vi "poll spawned task.vi"(0 "JSON string in":string, 5 "polling control":T1={"Timeout, ms (-1)"=-1, "polling period (ms)"={"starting"=4, "final"=128}, "interrupt polling notifier"=refnum}, 11 "error in (no error)":errorcluster) -> (3 "timeout?":bool, 4 "JSON received":string, 6 "Notifier out":refnum<notifier>, 8 "done":bool, 10 "Jl Server state out":T2, 12 "detailed error info":T3, 13 "Notification out":bool, 14 "return code":u8, 15 "error out":errorcluster)   [LabVIEW 2018, in "LV2Julia_core.lvlib"]
uses:
  LV2Julia_core.lvlib
  detailed error info.ctl
  StackFrame.ctl
  Server or client state.ctl
  polling control.ctl
  958caf3f-946f-4dc4-9902-e12cbf4cba19.vi
  958caf3f-946f-4dc4-9902-e12cbf4cba19.vi/ee613294-7676-459b-bae0-527ec17cd08f.vi
  958caf3f-946f-4dc4-9902-e12cbf4cba19.vi/ee613294-7676-459b-bae0-527ec17cd08f.vi/324bc100-61cc-4399-8a28-7e417bd8f265.vi
  958caf3f-946f-4dc4-9902-e12cbf4cba19.vi/ee613294-7676-459b-bae0-527ec17cd08f.vi/1a2262df-f044-41fe-b48a-3393a41bf191.vi
  958caf3f-946f-4dc4-9902-e12cbf4cba19.vi/ee613294-7676-459b-bae0-527ec17cd08f.vi/0df26e2a-8cb6-4a42-a810-c7ba34c0704a.vi
  check ID validity.vi
  bindata_descr to JSON.vi
  check cluster field names.vi
  concat JSON.vi
  build request.vi
  REQ full lifecycle.vi
  Parse server response.vi
  log jl exceptions.vi
panel:
  out "parsed response":cluster{"ticket":i32}
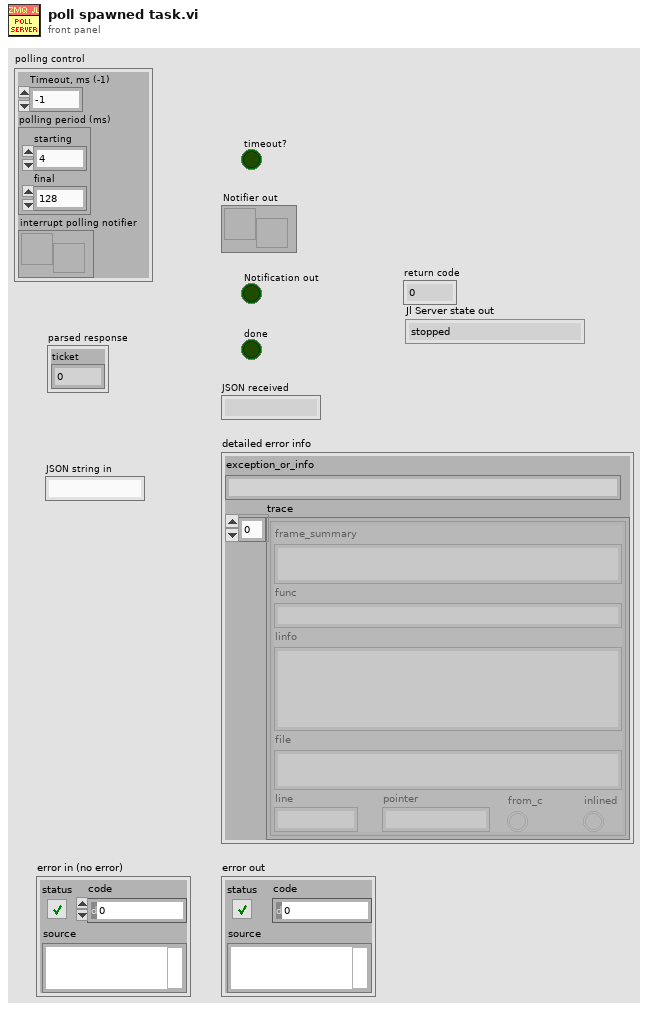
[diagram p1: front panel]
types:
  T1 = typedef "polling control.ctl" = cluster{"Timeout, ms (-1)":i32, "polling period (ms)":cluster{"starting":i32, "final":i32}, "interrupt polling notifier":refnum<notifier>}
  T2 = typedef "LV2Julia_core.lvlib/Server or client state.ctl" = enum16{"stopped", "running", "unknown"}
  T3 = typedef "LV2Julia_core.lvlib/detailed error info.ctl" = cluster{"exception_or_info":string, "trace":T4[]}
  T4 = typedef "LV2Julia_core.lvlib/StackFrame.ctl" = cluster{"frame_summary":string, "func":string, "linfo":string, "file":string, "line":i32, "pointer":u64, "from_c":bool, "inlined":bool}
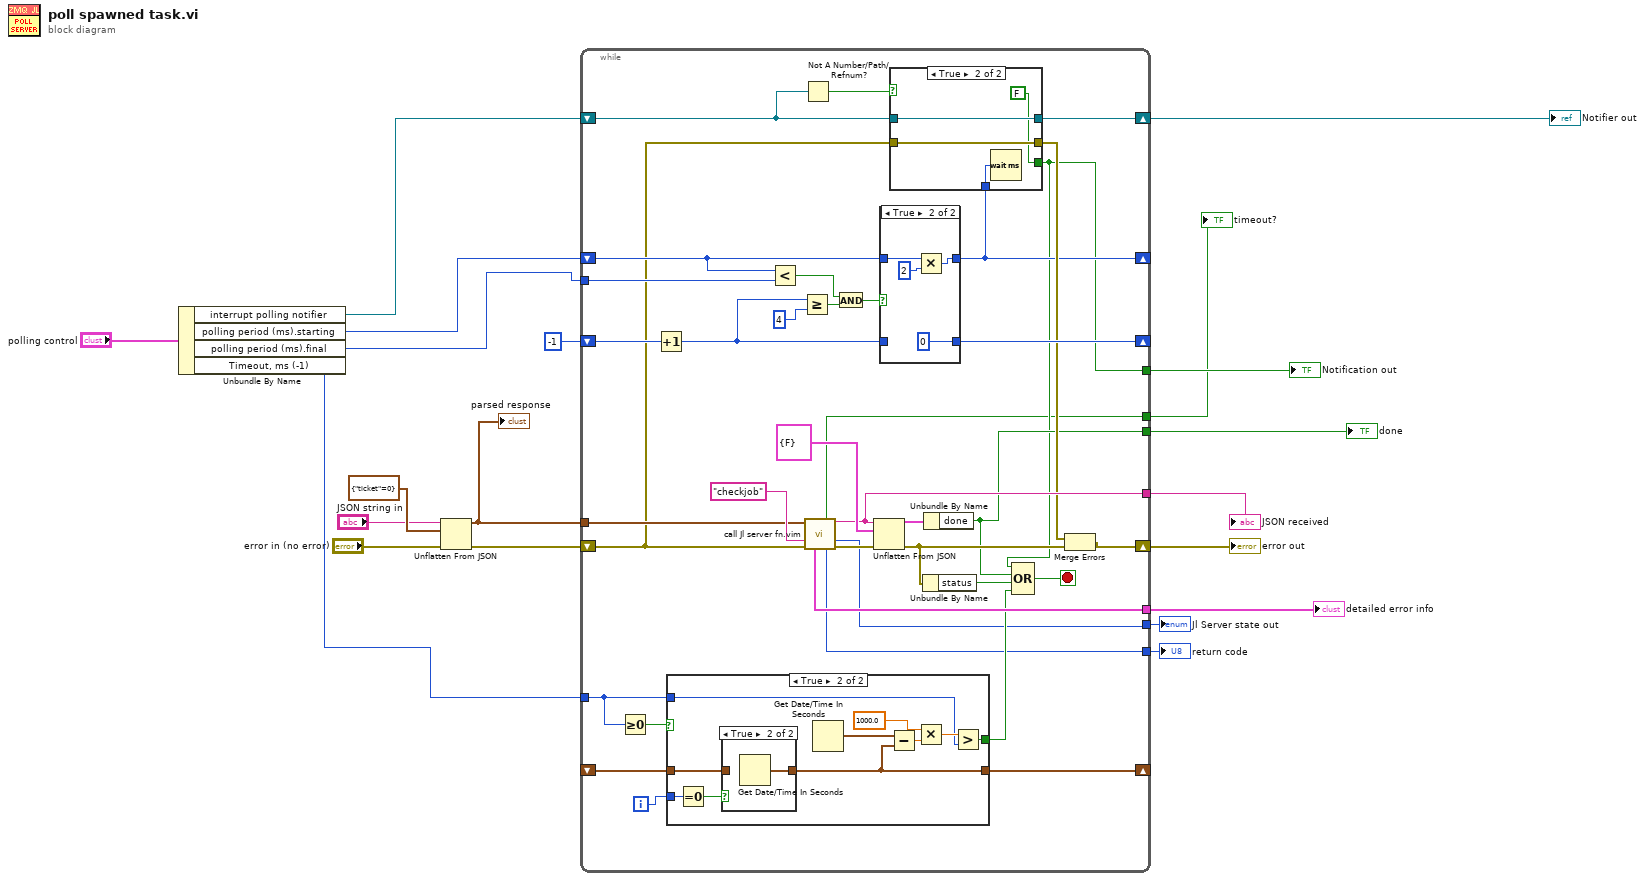
[diagram p0: block diagram]
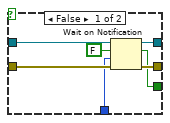
[diagram p2: hidden frame]
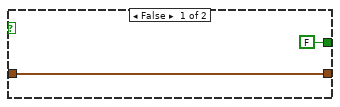
[diagram p3: hidden frame]
diagram:
  n1 = Unbundle By Name("polling control") -> ("interrupt polling notifier"=w1:refnum<notifier>, "polling period (ms).starting"=w3:i32, "polling period (ms).final"=w2:i32, "Timeout, ms (-1)"=w4:i32)
  n2 = Unflatten From JSON(JSON string="JSON string in", type and defaults=cluster{"ticket":i32} {"ticket"=0} ("parsed response"), error in (no error)="error in (no error)") -> (value=w6:cluster{"ticket":i32}, error out=w7:errorcluster)  [unwired: 4 in]
  "parsed response" <- w6
  n3 = while {
    tunnel: w6 -> [w56]
    tunnel: [w52] -> w13
    shift-right: [w38] -> w14
    shift-left: w7 -> [w39]
    shift-right: [w35] -> _
    shift-left: w3 -> [w42]
    shift-right: [w47] -> _
    shift-left: -1 ("counter") -> [w48]
    tunnel: w2 -> [w44]
    shift-right: [w36] -> w16
    shift-left: w1 -> [w21]
    tunnel: [w28] -> w20
    tunnel: w4 -> [w25]
    shift-right: [w30] -> _
    shift-left: _ -> [w33]
    tunnel: [w32] -> w17
    tunnel: [w31] -> w18
    tunnel: [w27] -> w19
    tunnel: [w24] -> w12
    tunnel: [w23] -> w11
    i -> [w34]
    stop <- w50 stop-if-true
    n4 = Greater Or Equal To 0?(x=w25) -> (x >= 0?=w26:bool)
    n5 = Increment(x=w48) -> (x+1=w41:i32)
    n6 = case shown="True" w26 {
      tunnel: w34 -> [_ w80]
      tunnel: w33 -> [w70 w78]
      tunnel: [w70 w76] -> w30
      tunnel: w25 -> [_ w72]
      tunnel: [FALSE w71] -> w29
      frame False {
      }
      frame True {
        n7 = Equal To 0?(x=w80) -> (x = 0?=w79:bool)
        n8 = case shown="True" w79 {
          tunnel: [w81 w82] -> w76
          tunnel: w78 -> [w81 _]
          frame False {
          }
          frame True {
            n9 = Get Date/Time In Seconds() -> (seconds since 1Jan1904=w82:timestamp)
          }
        }
        n10 = Get Date/Time In Seconds() -> (seconds since 1Jan1904=w77:timestamp)
        n11 = Subtract(x=w77, y=w76) -> (x-y=w75:dbl)
        n12 = Multiply(x=1000.0, y=w75) -> (x*y=w73:dbl)
        n13 = Greater?(x=w73, y=w72) -> (0:w71:bool)
      }
    }
    n14 = Less?(x=w42, y=w44) -> (x < y?=w43:bool)
    n15 = Greater Or Equal?(x=w41, y=4) -> (x >= y?=w45:bool)
    n16 = Not A Number/Path/Refnum?(number/path/refnum=w21) -> (NaN/Path/Refnum?=w22:bool)
    n17 = call "call Jl server fn.vim"("Arguments 1"=w56, "fun2call"="checkjob" ("Julia function name"), "error in (no error)"=w39) -> ("timeout?"=w27:bool, "JSON received"=w52:string, "Jl Server state out"=w23:T2, "detailed error info"=w31:T3, "return code"=w24:u8, "error out"=w55:errorcluster)  [unwired: 6 in, 1 out]
    n18 = And(x=w43, y=w45) -> (x .and. y?=w40:bool)
    n19 = Unflatten From JSON(JSON string=w52, type and defaults=cluster{"done":bool} {"done"=FALSE}, error in (no error)=w55) -> (value=w53:cluster{"done":bool}, error out=w51:errorcluster)  [unwired: 4 in]
    n20 = case shown="True" w40 {
      tunnel: w41 -> [w84 _]
      tunnel: [w84 0] -> w47
      tunnel: w42 -> [w83 w87]
      tunnel: [w83 w86] -> w35
      frame False {
      }
      frame True {
        n21 = Multiply(x=w87, y=2) -> (x*y=w86:i32)
      }
    }
    n22 = case shown="True" w22 {
      tunnel: w21 -> [w64 w66]
      tunnel: w39 -> [w63 w67]
      tunnel: [w62 w67] -> w37
      tunnel: [w61 w66] -> w36
      tunnel: w35 -> [w60 w68]
      tunnel: [w58 FALSE] -> w28
      frame False {
        n23 = Wait on Notification(notifier=w64, ignore previous (F)=FALSE, timeout in ms (-1)=w60, error in (no error)=w63) -> (notifier out=w61:refnum<notifier>, notification=w58:bool, error out=w62:errorcluster)  [unwired: 1 out]
      }
      frame True {
        n24 = Wait (ms)(milliseconds to wait=w68) -> ()  [unwired: 1 out]
      }
    }
    n25 = Unbundle By Name(w51) -> ("status"=w49:bool)
    n26 = Unbundle By Name(w53) -> ("done"=w32:bool)
    n27 = Compound Arithmetic op=OR(w28, w32, w49, w29) -> (w50:bool)
    n28 = Merge Errors(w37, w51) -> (w38:errorcluster)
  }
  "Notification out" <- w20
  "timeout?" <- w19
  "detailed error info" <- w18
  "done" <- w17
  "Notifier out" <- w16
  "error out" <- w14
  "JSON received" <- w13
  "return code" <- w12
  "Jl Server state out" <- w11
